vi "findSpeed.vi"() -> ()   [LabVIEW 2012]
panel:
  in  "Joystick 2x":dbl
  in  "Joystick 1X":dbl
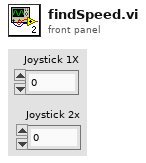
[diagram p1: front panel]
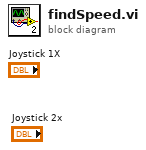
[diagram p0: block diagram]
diagram:
